vi "run.vi"(11 "function task in":refnum<class "function task.lvclass">) -> (2 "result":refnum<class "result.lvclass">, 3 "function task out":refnum<class "function task.lvclass">)   [LabVIEW 2013, in "function task.lvclass"]
uses:
  function task.lvclass
  result/result.lvclass
  task/task.lvclass
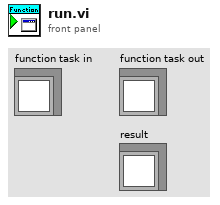
[diagram p1: front panel]
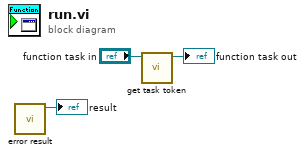
[diagram p0: block diagram]
diagram:
  n1 = call "error result.vi"() -> ("result"=→"result":refnum<class "result.lvclass">)  [unwired: 11 in]
  n2 = call "get task token.vi"("task in"="function task in") -> ("task out"=→"function task out":refnum<class "function task.lvclass">)  [unwired: 9 in, 1 out]
